vi "Read Device State Information Msg.vi"(11 "EMS Generic":refnum<class "EMS Generic.lvclass">) -> (2 "Return Device State Information Msg":refnum<class "Device State Information Msg.lvclass">, 3 "dup EMS Generic":refnum<class "EMS Generic.lvclass">)   [LabVIEW 2018, in "EMS Generic Actor.lvlib" / "EMS Generic.lvclass"]
uses:
  EMS Generic.lvclass
  EMS Generic Messages/Device State Information Msg/Device State Information Msg.lvclass
  EMS Generic.lvclass/EMS Generic.ctl
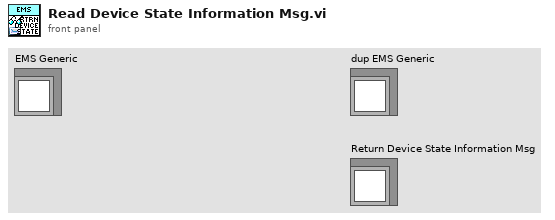
[diagram p1: front panel]
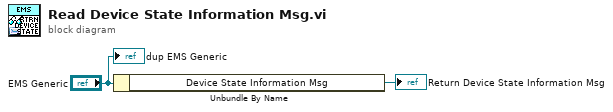
[diagram p0: block diagram]
diagram:
  n1 = Unbundle By Name("EMS Generic") -> ("Device State Information Msg"=→"Return Device State Information Msg":refnum<class "Device State Information Msg.lvclass">)
  "dup EMS Generic" <- "EMS Generic"
